vi "create daemon config.vi"(8 "error in (no error)":errorcluster) -> (0 "error out":errorcluster)   [LabVIEW 2016, in "update.lvlib"]
uses:
  update.lvlib
  <vilib>/Utility/config.llb/Write Key (String).vi
  <vilib>/Utility/config.llb/NI_LVConfig.lvlib
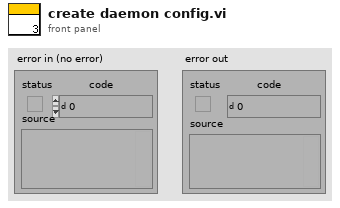
[diagram p1: front panel]
types:
  T1 = typedef "NI_LVConfig.lvlib/Config Data RefNum.ctl" = refnum<k1>
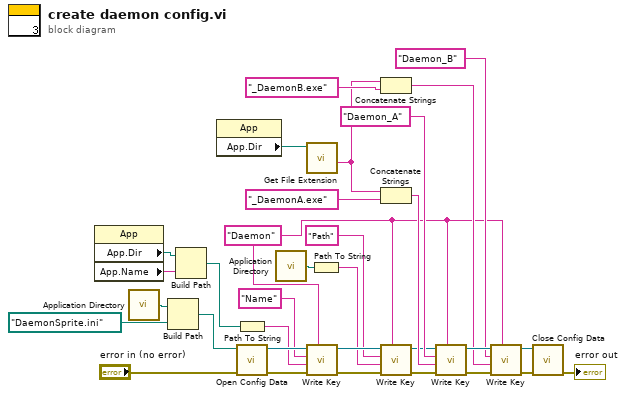
[diagram p0: block diagram]
diagram:
  w10 = "Daemon" ("section")
  n1 = property class="App"() -> ("App.Dir"=w5:path, "App.Name"=w4:string)  [unwired: 2 in, 2 out]
  n2 = call <vilib>:"Application Directory.vi"() -> ("Application Directory"=w32:path)
  n3 = Build Path(base path=w32, name or relative path=path "DaemonSprite.ini" ("Application Directory")) -> (appended path=w31:path)
  n4 = Build Path(base path=w5, name or relative path=w4) -> (appended path=w3:path)
  n5 = property class="App"() -> ("App.Dir"=w25:path)  [unwired: 2 in, 2 out]
  n6 = Path To String(path=w3) -> (string=w2:string)
  n7 = call <vilib>:"Open Config Data.vi"("error in (no error)"="error in (no error)", "configuration file path"=w31) -> ("error out"=w15:errorcluster, "refnum"=w14:T1)  [unwired: 7 in, 1 out]
  n8 = call <vilib>:"Application Directory.vi"() -> ("Application Directory"=w8:path)
  n9 = call <vilib>:"Get File Extension.vi"("file"=w25) -> ("filename without extension"=w23:string)  [unwired: 6 in, 4 out]
  n10 = call-poly <vilib>:"Write Key.vi"("section"=w10, "error in (no error)"=w15, "value"=w2, "key"="Name", "refnum"=w14) -> ("error out"=w12:errorcluster, "refnum out"=w11:T1)  [unwired: 4 in, 1 out]
  n11 = Path To String(path=w8) -> (string=w1:string)
  n12 = Concatenate Strings(w23, "_DaemonB.exe" ("名称或相对路径")) -> (w21:string)
  n13 = Concatenate Strings(w23, "_DaemonA.exe" ("名称或相对路径")) -> (w22:string)
  n14 = call-poly <vilib>:"Write Key.vi"("section"=w10, "error in (no error)"=w12, "value"=w1, "key"="Path", "refnum"=w11) -> ("error out"=w6:errorcluster, "refnum out"=w7:T1)  [unwired: 4 in, 1 out]
  n15 = call-poly <vilib>:"Write Key.vi"("section"=w10, "error in (no error)"=w6, "value"=w22, "key"="Daemon_A", "refnum"=w7) -> ("error out"=w29:errorcluster, "refnum out"=w30:T1)  [unwired: 4 in, 1 out]
  n16 = call-poly <vilib>:"Write Key.vi"("section"=w10, "error in (no error)"=w29, "value"=w21, "key"="Daemon_B", "refnum"=w30) -> ("error out"=w18:errorcluster, "refnum out"=w17:T1)  [unwired: 4 in, 1 out]
  n17 = call <vilib>:"Close Config Data.vi"("error in (no error)"=w18, "refnum"=w17) -> ("error out"=→"error out":errorcluster)  [unwired: 8 in, 1 out]
